vi "Set Channels Buffer.vi"(10 "channels buffer":dbl[](array[numeric]), 11 "Transceiver Thread in":refnum<class "Plugin Thread.lvclass">) -> (3 "Transceiver Thread out":refnum<class "Plugin Thread.lvclass">)   [LabVIEW 2017, in "DSF Core.lvlib" / "Plugin Thread.lvclass"]
uses:
  Plugin Thread.lvclass
  Plugin Thread.lvclass/Plugin Thread.ctl
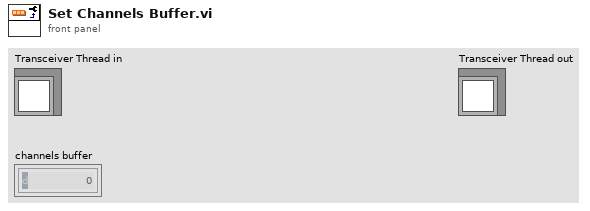
[diagram p1: front panel]
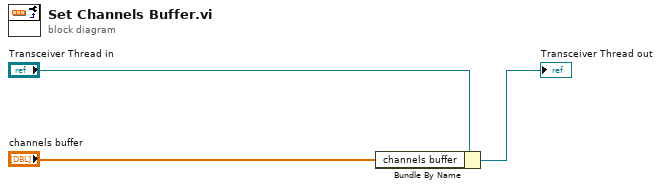
[diagram p0: block diagram]
diagram:
  n1 = Bundle By Name(cluster="Transceiver Thread in", "channels buffer"="channels buffer") -> (→"Transceiver Thread out":refnum<class "Plugin Thread.lvclass">)
